vi "Translate_PolarVector.vi"(7 "Translation Type":T1, 8 "error in (no error)":errorcluster, 10 "PolarVector.lvclass":refnum<class "PolarVector.lvclass">, 11 "CartesianVector in":refnum<class "CartesianVector.lvclass">) -> (0 "error out":errorcluster, 3 "CartesianVector out":refnum<class "CartesianVector.lvclass">)   [LabVIEW 2011, in "CartesianVector.lvclass"]
doc: "Translates a CartesianVector object either additively or subtractively by a PolarVector object. Outputs a new CartesianVector object that has been translated."
uses:
  CartesianVector.lvclass
  TypeDefs/TranslationType.ctl
  PolarVector/PolarVector.lvclass
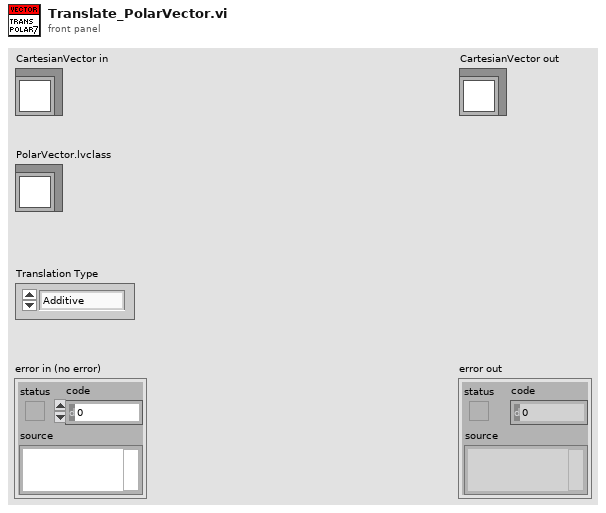
[diagram p1: front panel]
types:
  T1 = typedef "TranslationType.ctl" = enum16{"Additive", "Subtractive"}
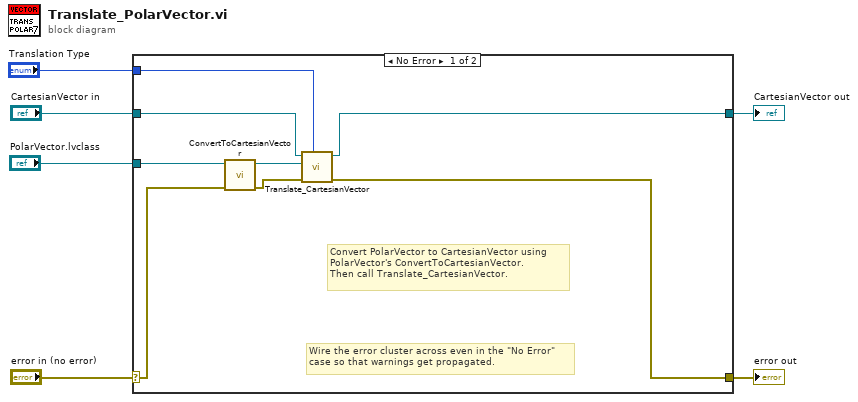
[diagram p0: block diagram]
diagram:
  n1 = case shown="No Error" "error in (no error)" {
    selector: "error in (no error)" -> [w9 w16]
    tunnel: [w7 w16] -> w5
    tunnel: [w10 w15] -> w3
    tunnel: "CartesianVector in" -> [w12 w15]
    tunnel: "PolarVector.lvclass" -> [w14 _]
    tunnel: "Translation Type" -> [w11 _]
    frame No Error {
      # "Convert PolarVector to CartesianVector using\nPolarVector's ConvertToCartesianVector.\nThen call Translate_CartesianVector."
      # "Wire the error cluster across even in the \"No Error\"\ncase so that warnings get propagated."
      n2 = call "ConvertToCartesianVector.vi"("error in (no error)"=w9, "PolarVector in"=w14) -> ("error out"=w8:errorcluster, "CartesianVector.lvclass"=w13:refnum<class "CartesianVector.lvclass">)  [unwired: 8 in]
      n3 = call "Translate_CartesianVector.vi"("Translation Type"=w11, "error in (no error)"=w8, "CV 2"=w13, "CV 1"=w12) -> ("error out"=w7:errorcluster, "CV 1 Translated by CV 2"=w10:refnum<class "CartesianVector.lvclass">)  [unwired: 6 in]
    }
    frame Error {
    }
  }
  "error out" <- w5
  "CartesianVector out" <- w3
